vi "pid.vi"(4 "y":dbl, 6 "Te":dbl=0.05, 7 "Kp":dbl=0.4, 9 "r - Set point":dbl=55.0, 10 "Kd":dbl=0.1, 11 "Ki":dbl=0.9) -> (3 "u":dbl)   [LabVIEW 2020]
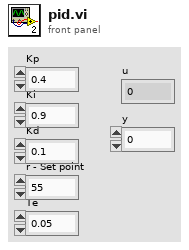
[diagram p1: front panel]
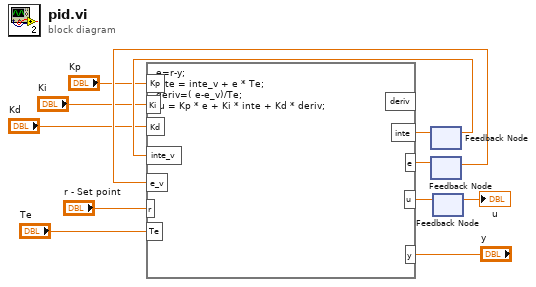
[diagram p0: block diagram]
diagram:
  n1 = feedback #1() -> (w9:dbl)  [unwired: 1 in]
  n2 = feedback #2() -> (w11:dbl)  [unwired: 1 in]
  n3 = formula code="e=r-y;\ninte = inte_v + e * Te;\nderiv=( e-e_v)/Te;\n u = Kp * e + Ki * inte + Kd * deriv;"("inte_v"=w9, "Te"="Te", "e_v"=w11, "Kp"="Kp", "Ki"="Ki", "Kd"="Kd", "r"="r - Set point", "y"="y") -> ("inte"=w8:dbl, "u"=w4:dbl, "e"=w10:dbl)  [unwired: 1 out]
  n4 = feedback-in #1(w8) -> ()
  n5 = feedback-in #2(w10) -> ()
  n6 = feedback #3() -> (→"u":dbl)  [unwired: 1 in]
  n7 = feedback-in #3(w4) -> ()
